vi "UI_History.vi"() -> ()   [LabVIEW 2014]
panel:
  out "结果":u32
  in  "查询":bool
  in  "选项卡控件":enum32{"陪试轴承单元", "试验轴承单元", "加载单元", "主轴监测单元"}(tab)
  out "出油温度2":dbl[](graph)
  out "出油温度1":dbl[](graph)
  out "摩擦力矩":dbl[](graph)
  out "出油温度":dbl[](graph)
  out "轴承外圈温度":dbl[](graph)
  out "外壳振动1":dbl[](graph)
  out "外壳振动2":dbl[](graph)
  out "轴向油缸力":dbl[](graph)
  out "径向油缸力":dbl[](graph)
  out "径向位移SRR2":dbl[](graph)
  out "径向位移SRR1":dbl[](graph)
  out "径向位移SLR2":dbl[](graph)
  out "径向位移SLR1":dbl[](graph)
  out "轴向位移SA":dbl[](graph)
  out "转速":cluster{"X":dbl, "Y":dbl}[](graph)
  in  "下拉列表":u16(ring) items=["陪试轴承单元", "试验轴承单元", "加载单元", "主轴监测单元"]
  in  "结束时间":timestamp
  in  "开始时间":timestamp
  # "历史信息"
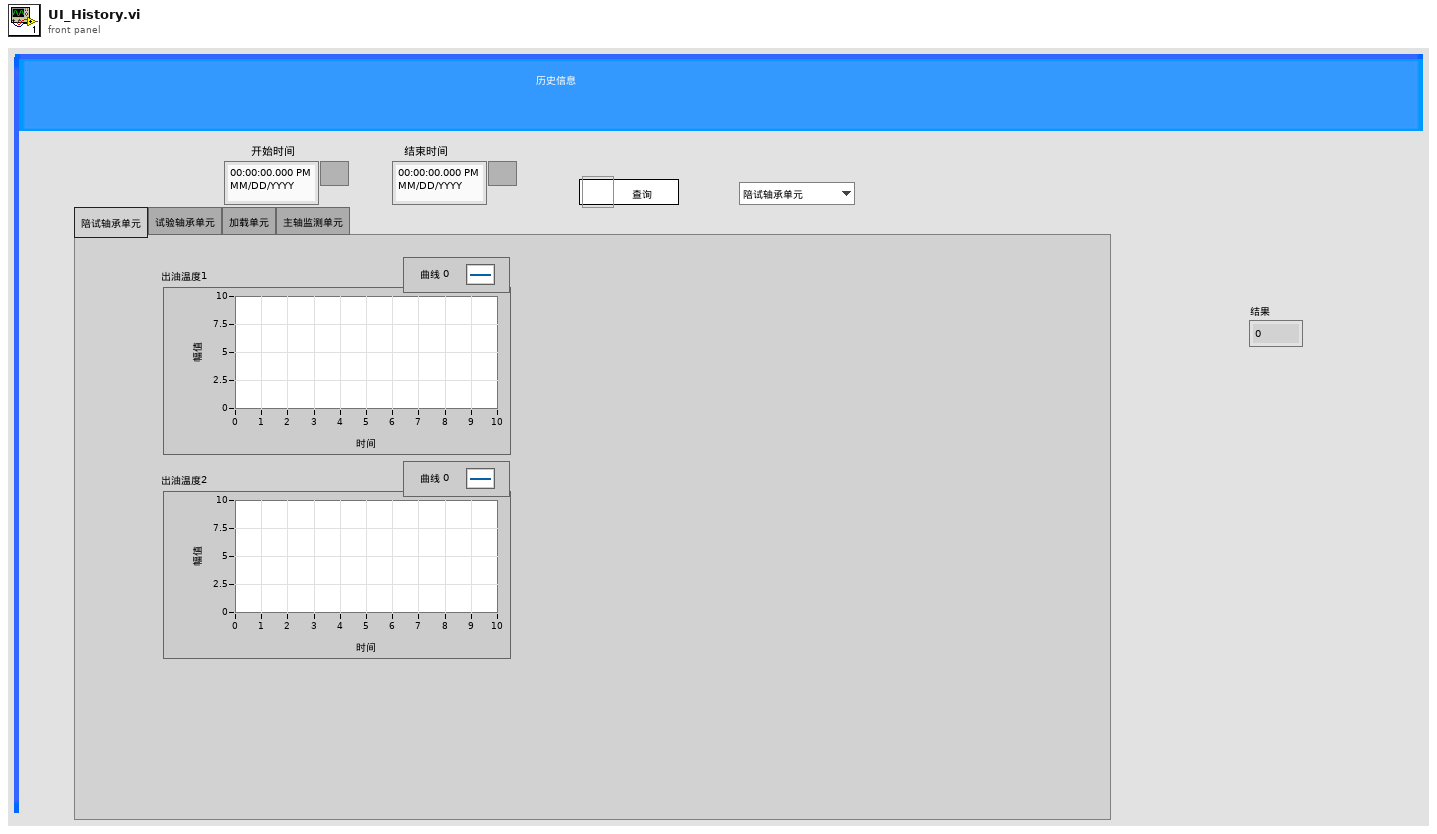
[diagram p1: front panel]
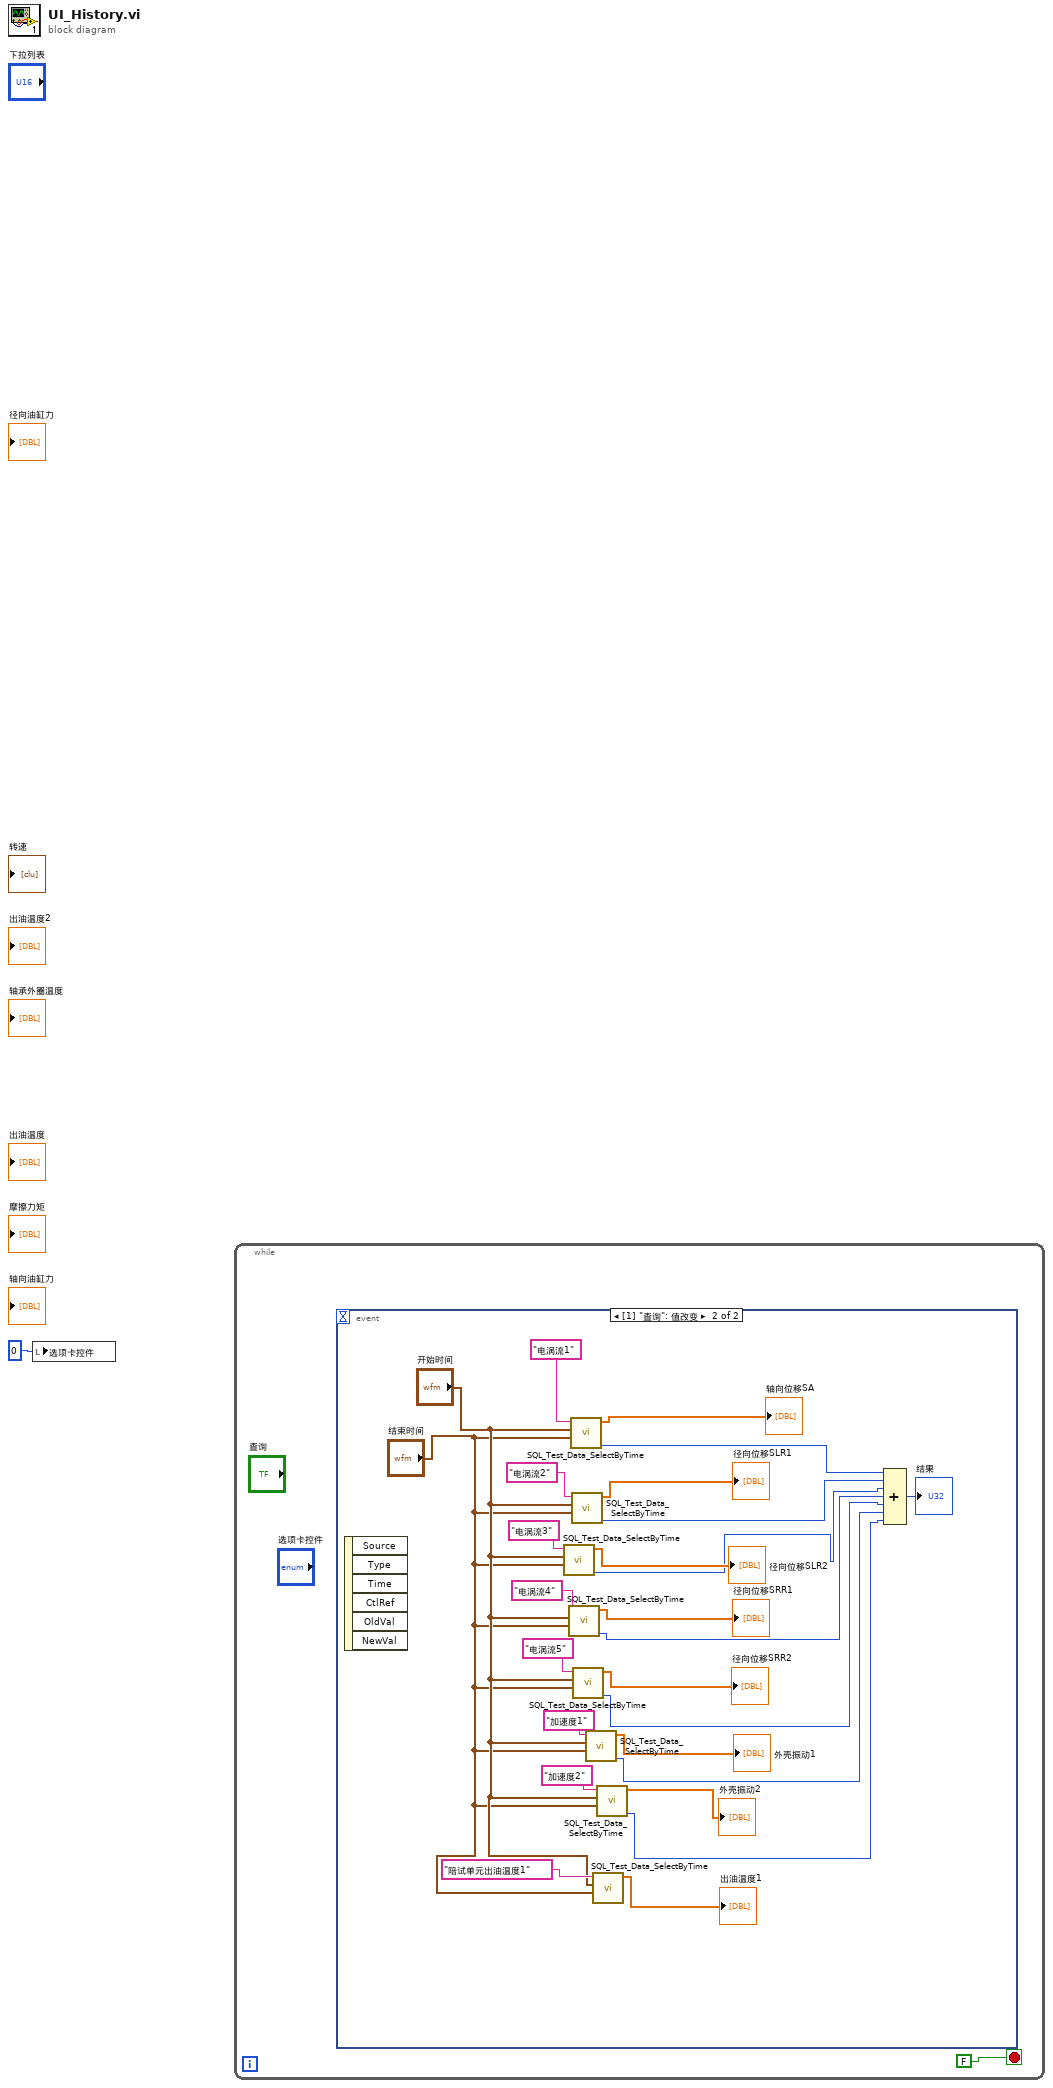
[diagram p0: block diagram]
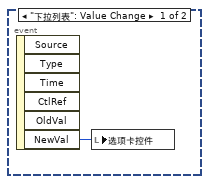
[diagram p2: hidden frame]
diagram:
  n1 = local write "选项卡控件"(0) -> ()
  n2 = while {
    stop <- FALSE stop-if-true
    n3 = event shown="[1] \"查询\": 值改变" {
      selector: _ -> [_ _]
      dyn-events: _ -> [_ _]
      timeout: _ -> [_ _]
      event "下拉列表": Value Change {
        n4 = event-data() -> ("NewVal"=w3:u16)  [unwired: 1 in, 5 out]
        n5 = local write "选项卡控件"(w3) -> ()
      }
      event "查询": Value Change {
        n6 = event-data() -> ()  [unwired: 1 in, 6 out]
        n7 = call "SQL_Test_Data_SelectByTime.vi"("结束时间"="结束时间", "起始时间"="开始时间", "通道名"="电涡流3") -> ("x-y"=w8:u32, "数据"=→"径向位移SLR2":dbl[])  [unwired: 4 in, 1 out]
        n8 = call "SQL_Test_Data_SelectByTime.vi"("结束时间"="结束时间", "起始时间"="开始时间", "通道名"="电涡流4") -> ("x-y"=w20:u32, "数据"=→"径向位移SRR1":dbl[])  [unwired: 4 in, 1 out]
        n9 = call "SQL_Test_Data_SelectByTime.vi"("结束时间"="结束时间", "起始时间"="开始时间", "通道名"="电涡流1") -> ("x-y"=w22:u32, "数据"=→"轴向位移SA":dbl[])  [unwired: 4 in, 1 out]
        n10 = call "SQL_Test_Data_SelectByTime.vi"("结束时间"="结束时间", "起始时间"="开始时间", "通道名"="电涡流2") -> ("x-y"=w21:u32, "数据"=→"径向位移SLR1":dbl[])  [unwired: 4 in, 1 out]
        n11 = call "SQL_Test_Data_SelectByTime.vi"("结束时间"="结束时间", "起始时间"="开始时间", "通道名"="电涡流5") -> ("x-y"=w19:u32, "数据"=→"径向位移SRR2":dbl[])  [unwired: 4 in, 1 out]
        n12 = call "SQL_Test_Data_SelectByTime.vi"("结束时间"="结束时间", "起始时间"="开始时间", "通道名"="加速度1") -> ("x-y"=w18:u32, "数据"=→"外壳振动1":dbl[])  [unwired: 4 in, 1 out]
        n13 = call "SQL_Test_Data_SelectByTime.vi"("结束时间"="结束时间", "起始时间"="开始时间", "通道名"="陪试单元出油温度1") -> ("数据"=→"出油温度1":dbl[])  [unwired: 4 in, 2 out]
        n14 = call "SQL_Test_Data_SelectByTime.vi"("结束时间"="结束时间", "起始时间"="开始时间", "通道名"="加速度2") -> ("x-y"=w17:u32, "数据"=→"外壳振动2":dbl[])  [unwired: 4 in, 1 out]
        n15 = Compound Arithmetic op=ADD(w22, w21, w8, w20, w19, w18, w17) -> (→"结果":u32)
      }
    }
  }
